vi "Init fp settings.vi"(6 "error in (no error)":errorcluster, 7 "Enable Modal (T)":bool=TRUE, 8 "Caller VI Refnum (Callee's Caller)":refnum<vi>, 9 "vi reference":refnum<vi>) -> (0 "error out":errorcluster, 3 "vi reference out":refnum<vi>, 4 "Front Panel Window:Panel Bounds":T2, 5 "Original basic fp settings":T1)   [LabVIEW 2020]
uses:
  <vilib>/Utility/miscctls.llb/LVRectTypeDef.ctl
  Basic FP Settings--cluster.ctl
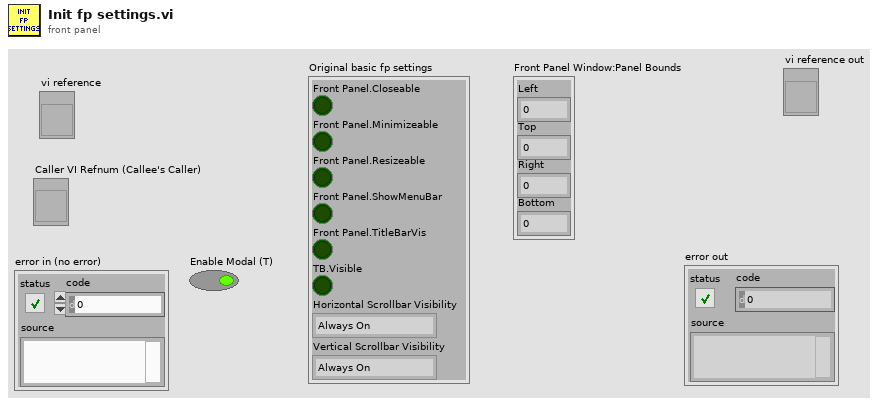
[diagram p1: front panel]
types:
  T1 = typedef "Basic FP Settings--cluster.ctl" = cluster{"Front Panel.Closeable":bool, "Front Panel.Minimizeable":bool, "Front Panel.Resizeable":bool, "Front Panel.ShowMenuBar":bool, "Front Panel.TitleBarVis":bool, "TB.Visible":bool, "Horizontal Scrollbar Visibility":enum16{"Always On", "Always Off", "Off While Running"}, "Vertical Scrollbar Visibility":enum16{"Always On", "Always Off", "Off While Running"}}
  T2 = typedef "LVRectTypeDef.ctl" = cluster{"Left":i16, "Top":i16, "Right":i16, "Bottom":i16}
  T3 = enum16{"Always On", "Always Off", "Off While Running"}
  T4 = enum32{"Invalid", "Default", "Floating", "Floating/Auto-Hide", "Modal"}
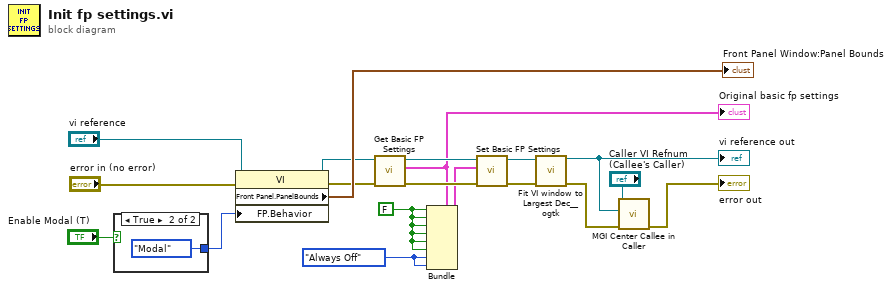
[diagram p0: block diagram]
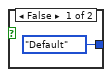
[diagram p2: hidden frame]
diagram:
  w15 = T3."Always Off" ("Horizontal Scrollbar Visibility")
  w16 = FALSE ("Front Panel.Closeable")
  n1 = case shown="True" "Enable Modal (T)" {
    tunnel: [T4."Default" ("Front Panel Window:Behavior") T4."Modal" ("Front Panel Window:Behavior")] -> w13
    frame False {
    }
    frame True {
    }
  }
  n2 = property class="VI"(reference="vi reference", error in="error in (no error)", "FP.Behavior"=w13) -> (reference out=w10:refnum<vi>, error out=w11:errorcluster, "Front Panel.PanelBounds"=→"Front Panel Window:Panel Bounds":T2)
  n3 = call "Get Basic FP Settings.vi"("error in (no error)"=w11, "vi reference"=w10) -> ("error out"=w19:errorcluster, "basic fp settings"=w17:T1, "vi reference out"=w18:refnum<vi>)  [unwired: 7 in]
  "Original basic fp settings" <- w17
  n4 = Bundle(cluster=w17, "Front Panel.Closeable"=w16, "Front Panel.Minimizeable"=w16, "Front Panel.Resizeable"=w16, "Front Panel.ShowMenuBar"=w16, "Front Panel.TitleBarVis"=w16, "TB.Visible"=w16, "Horizontal Scrollbar Visibility"=w15, "Vertical Scrollbar Visibility"=w15) -> (w14:T1)
  n5 = call "Set Basic FP Settings.vi"("error in (no error)"=w19, "basic fp settings"=w14, "vi reference"=w18) -> ("error out"=w8:errorcluster, "vi reference out"=w9:refnum<vi>)  [unwired: 7 in]
  n6 = call <userlib>:"Fit VI window to Largest Dec__ogtk.vi"("error in (no error)"=w8, "VI Ref (calling VI)"=w9) -> ("error out"=w6:errorcluster, "dup VI Ref"=w2:refnum<vi>)  [unwired: 4 in]
  "vi reference out" <- w2
  n7 = call <userlib>:"MGI Center Callee in Caller.vi"("Error In"=w6, "Callee VI Refnum (Caller)"=w2, "Caller VI Refnum (Callee's Caller)"="Caller VI Refnum (Callee's Caller)") -> ("Error Out"=→"error out":errorcluster)  [unwired: 8 in]
